vi "Convert U8x32 to U256.vi"(7 "U8x32":u8[](array[numeric])=[0, 0, 0, 0, 0, 0, 0, 0, 0, 0, 0, 0, 0, 0, 0, 0, 0, 0, 0, 0, 0, 0, 0, 0, 0, 0, 0, 0, 0, 0, 0, 0]) -> (8 "U64x4 CLuster":T1)   [LabVIEW 2012]
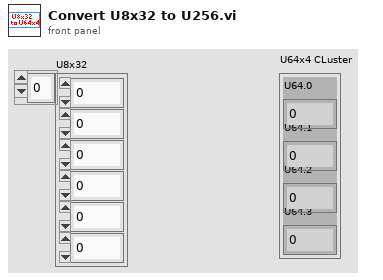
[diagram p1: front panel]
types:
  T1 = cluster{"U64.0":u64, "U64.1":u64, "U64.2":u64, "U64.3":u64}
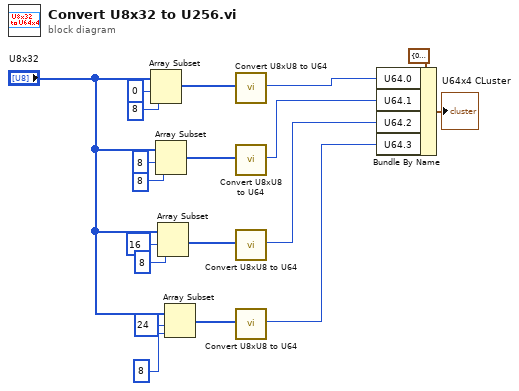
[diagram p0: block diagram]
diagram:
  n1 = Array Subset(array="U8x32", index=0, length=8) -> (w11:u8[])
  n2 = Array Subset(array="U8x32", index=8, length=8) -> (w10:u8[])
  n3 = Array Subset(array="U8x32", index=16, length=8) -> (w9:u8[])
  n4 = Array Subset(array="U8x32", index=24, length=8) -> (w8:u8[])
  n5 = call <userlib>:"Convert U8xU8 to U64.vi"("Input Data"=w11) -> ("U64"=w6:u64)  [unwired: 18 in]
  n6 = call <userlib>:"Convert U8xU8 to U64.vi"("Input Data"=w10) -> ("U64"=w5:u64)  [unwired: 18 in]
  n7 = call <userlib>:"Convert U8xU8 to U64.vi"("Input Data"=w9) -> ("U64"=w4:u64)  [unwired: 18 in]
  n8 = call <userlib>:"Convert U8xU8 to U64.vi"("Input Data"=w8) -> ("U64"=w3:u64)  [unwired: 18 in]
  n9 = Bundle By Name(cluster=T1 {"U64.0"=0, "U64.1"=0, "U64.2"=0, "U64.3"=0} ("Output Data"), "U64.0"=w6, "U64.1"=w5, "U64.2"=w4, "U64.3"=w3) -> (→"U64x4 CLuster":T1)
